vi "Return Msg.vi"(8 "error in (no error)":errorcluster, 11 "Panel Behavior.lvclass":refnum<class "Panel Behavior.lvclass">) -> (0 "error out":errorcluster, 2 "Console2API Q.lvclass":refnum<class "Console Reply.lvclass">, 3 "Panel Behavior.lvclass":refnum<class "Panel Behavior.lvclass">)   [LabVIEW 2015, in "EditPanel API.lvlib" / "Panel Behavior.lvclass"]
uses:
  Panel Behavior.lvclass
  Console Reply/Console Reply/Console Reply.lvclass
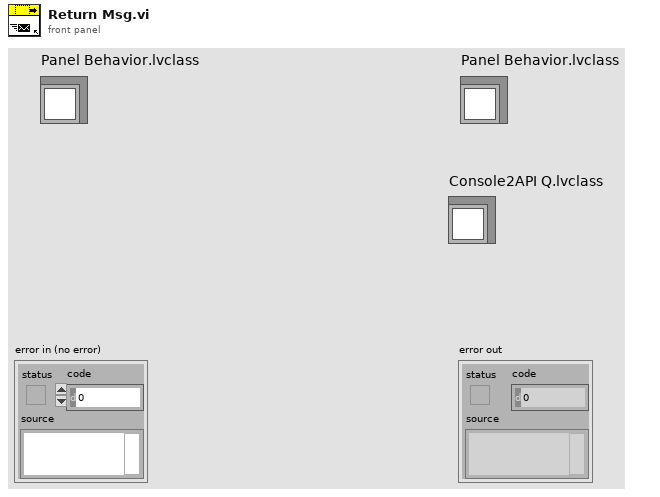
[diagram p1: front panel]
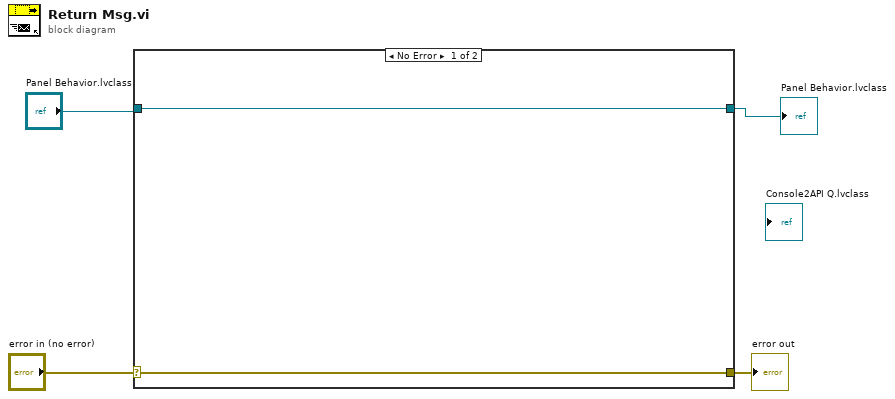
[diagram p0: block diagram]
diagram:
  n1 = case shown="No Error" "error in (no error)" {
    selector: "error in (no error)" -> [w5 w8]
    tunnel: [w5 w8] -> w3
    tunnel: [w6 w7] -> w1
    tunnel: "Panel Behavior.lvclass" -> [w6 w7]
    frame No Error {
    }
    frame Error {
    }
  }
  "error out" <- w3
  "Panel Behavior.lvclass" <- w1
